vi "System Subpanel.vi"() -> ()   [LabVIEW 2021, in "CIF Manager UI.lvlib"]
uses:
  CIF Manager UI.lvlib
  CIFManagerUI Class/Typedef/New Plugin.ctl
  CIFManagerUI Class/Typedef/Class Data for Manager SubPanel.ctl
  <vilib>/gRPC/LabVIEW gRPC Library/Shared/grpcId.ctl
  <vilib>/CIF Foundation/CIF Core/CIFUI/Typedef/Core UI References.ctl
  <vilib>/CIF Foundation/CIF Core/CIFUI/Typedef/Run Listen Button.ctl
  <vilib>/CIF Foundation/CIF Core/CIFUI/Typedef/SubPanel Events.ctl
  <vilib>/CIF Foundation/CIF Core/CIFUI/Typedef/New Connection Event Data.ctl
  <vilib>/CIF Foundation/CIF Core/CIFUI/Typedef/New Connection Plugin Event Data.ctl
  CIFManagerUI Class/Typedef/Core Manager UI References.ctl
  CIFManagerUI Class/Typedef/Channel Connection.ctl
  CIFManagerUI Class/Typedef/CIF_Manager_UI_Tab.ctl
  CIFManagerUI Class/CIF_Manager_UI.lvclass/CIF_Manager_UI.ctl
  <vilib>/CIF Foundation/CIF Core/CIFUI/CIF_UI.lvclass/CIF_UI.ctl
  <vilib>/CIF Foundation/CIF Core/CIFUI/Utilities/Get Human Readable Error.vi
  <vilib>/CIF Foundation/CIF Utilities/Errors/Append Error Location.vi
  <vilib>/CIF Foundation/CIF Core/CIFUI/Accessors/Read Instrument Studio.vi
  CIFManagerUI Class/CIF_Manager_UI.lvclass
  C:/Program Files/National Instruments/LabVIEW 2021/vi.lib/CIF Foundation/CIF Core/CIFUI/CIF_UI.lvclass
  <vilib>/CIF Foundation/CIF Core/CIFUI/UI Helpers/UI Element Update/Empty Tree by Reference.vi
  CIFManagerUI Class/Manager Functions/SubVIs/Initialize Manager Tab by Reference.vi
  <vilib>/CIF Foundation/CIF Utilities/Errors/Human Readable Error Message.vi
  <vilib>/CIF Foundation/CIF Core/CIFUI/CIF_UI.lvclass
  <vilib>/CIF Foundation/CIF Core/CIFPluginManager/gRPC/CIF_Manager_Client_Wrapper/CIFManagerClientWrapper.lvlib
  <vilib>/gRPC/LabVIEW gRPC Library/grpc-lvsupport-release.lvlib
panel:
  in  "Class Data for Manager SubPanel":T1
  in  "Update Plugin Types":bool
  in  "Load Plugin":bool
  in  "Reset Info":bool
  in  "Get All Info":bool
  in  "Discovered Plugins":string(tree)
  in  "Loaded Plugins":string(tree)
  in  "New Plugin":T6={"Unique Name"="test", "Type"="", "Version (Optional)"="", "Loader (Optional)"=""}
  in  "Abort Plugin":bool
  in  "Plugin to abort":string
  in  "Abort All Plugins":bool
  out "Plugin Metadata":string="\n\n\n\n\n\n\n\n\n\n\n\n\n\n\n\n\n\n\n\n\n\n\n"
  out "Info":string
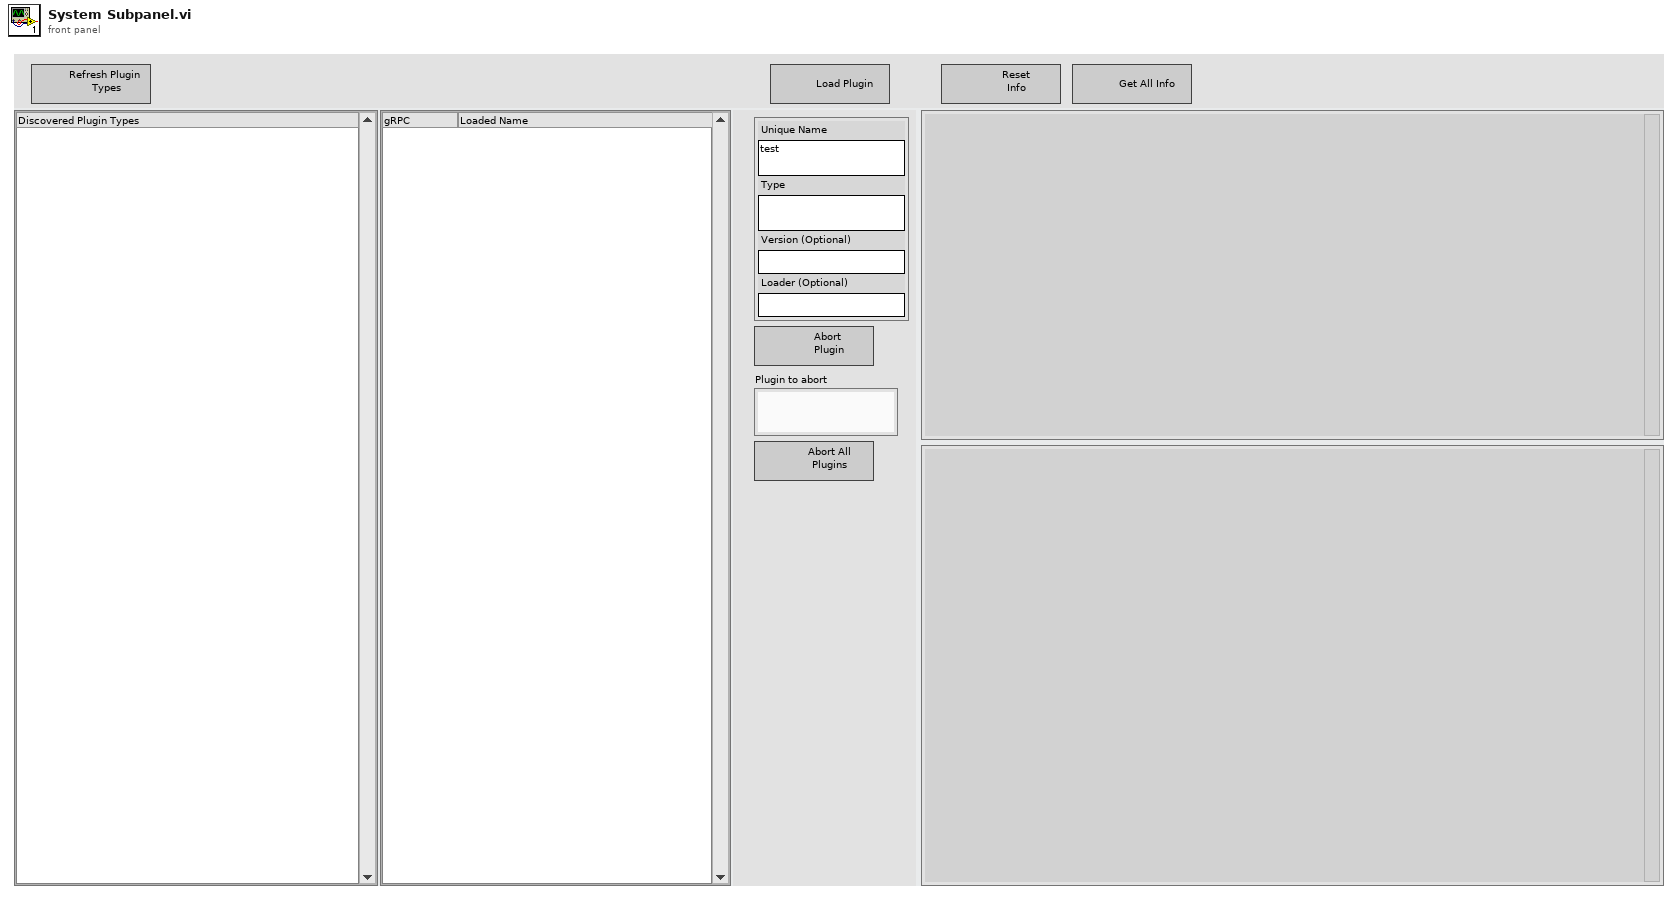
[diagram p1: front panel]
types:
  T1 = typedef "CIF_Manager_UI.lvclass/Class Data for Manager SubPanel.ctl" = cluster{"Class Data for SubPanel":cluster{"IP Address":string, "Manager gRPC ID":T2, "Server Certificate File (.crt)":path, "Connected":bool, "Manager Connection":bool, "Core UI References":T3, "Subpanel Events":T4}, "Manager UI References":T5}
  T2 = typedef "grpc-lvsupport-release.lvlib/grpcId.ctl" = u64
  T3 = typedef "CIF_UI.lvclass/Core UI References.ctl" = cluster{"Plugin Status":refnum<vi>, "Plugin Status Valid":bool, "Connection":refnum<vi>, "Connection Valid":bool, "Exit":refnum<vi>, "Exit Valid":bool, "Run Listen":refnum<vi>, "Run Listen Valid":bool, "Clear Local Error":refnum<vi>, "Clear Local Error Valid":bool, "Local Error":refnum<vi>, "Local Error Valid":bool}
  T4 = typedef "CIF_UI.lvclass/SubPanel Events.ctl" = cluster{"Clear Local Error":refnum<user-event>, "Shutdown":refnum<user-event>, "gRPC Connection":refnum<user-event>, "Plugin Connection":refnum<user-event>}
  T5 = typedef "CIF_Manager_UI.lvclass/Core Manager UI References.ctl" = cluster{"Discovered Plugins":refnum<vi>, "Discovered Plugins Valid":bool, "Loaded Plugins":refnum<vi>, "Loaded Plugins Valid":bool, "Publisher Channels":refnum<vi>, "Publisher Channels Valid":bool, "Subscriber Channels":refnum<vi>, "Subscriber Channels Valid":bool, "Channel Connection":refnum<vi>, "Channel Connection Valid":bool, "New Plugin Load":refnum<vi>, "New Plugin Load Valid":bool, "Errors":refnum<vi>, "Errors Valid":bool, "Plugin to Abort":refnum<vi>, "Plugin to Abort Valid":bool, "CIF Manager Tab":refnum<vi>, "Manger Tab Valid":bool, "System Errors":refnum<vi>, "System Errors Valid":bool, "Plugin Selection":refnum<vi>, "Plugin Selection Valid":bool}
  T6 = typedef "CIF_Manager_UI.lvclass/New Plugin.ctl" = cluster{"Unique Name":string, "Type":string, "Version (Optional)":string, "Loader (Optional)":string}
  T7 = typedef "CIF_Manager_client.lvlib/cif_management_common_PluginMetadata.ctl" = cluster{"description":string, "history":string, "author":string}
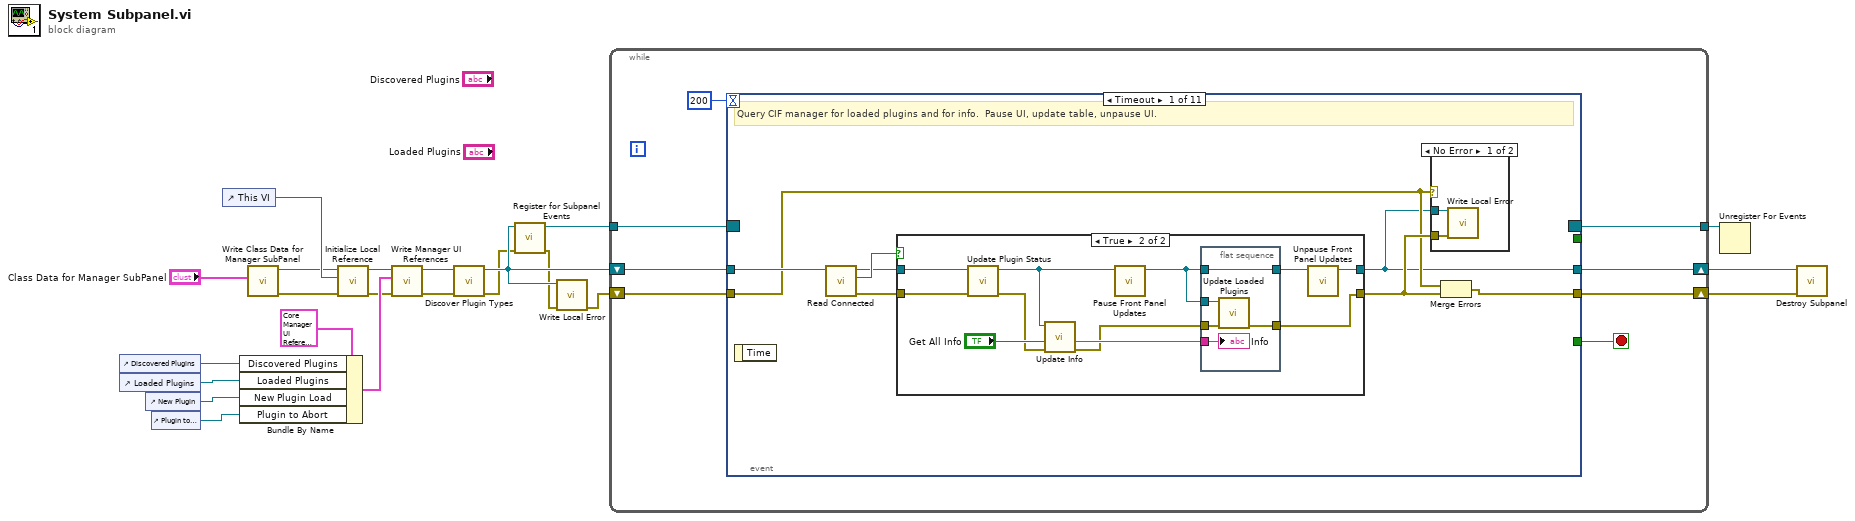
[diagram p0: block diagram]
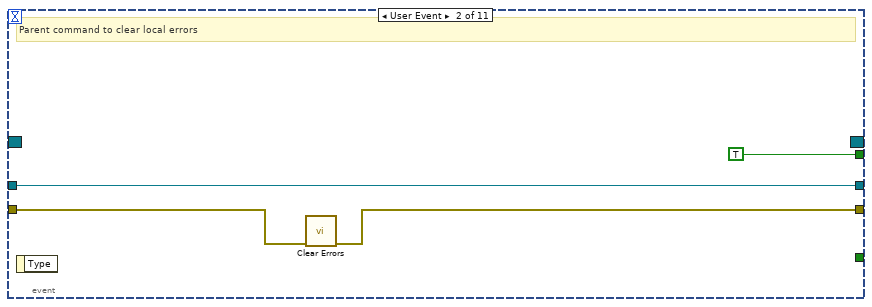
[diagram p4: hidden frame]
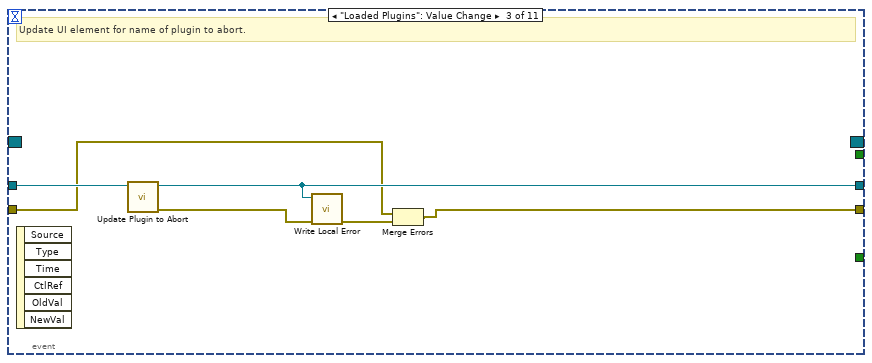
[diagram p5: hidden frame]
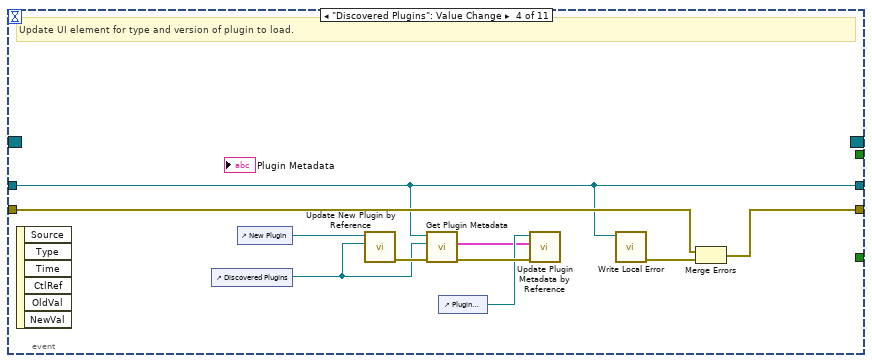
[diagram p6: hidden frame]
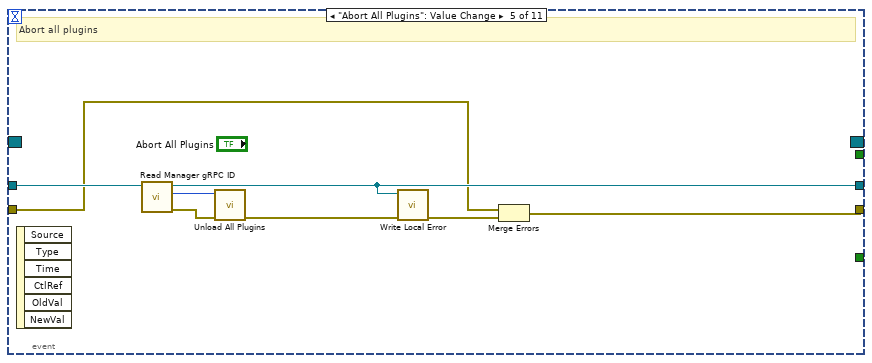
[diagram p7: hidden frame]
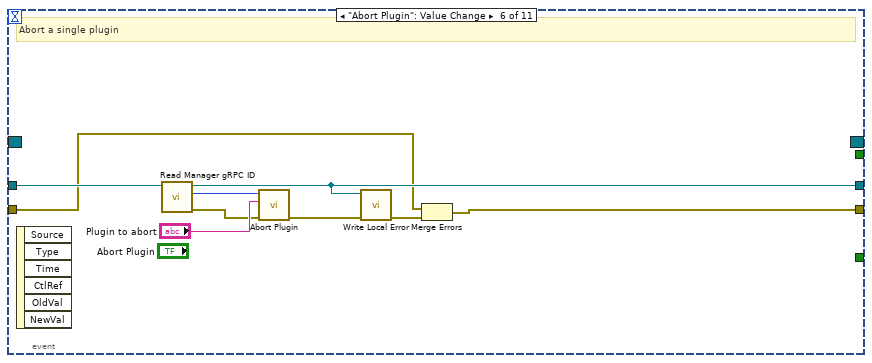
[diagram p8: hidden frame]
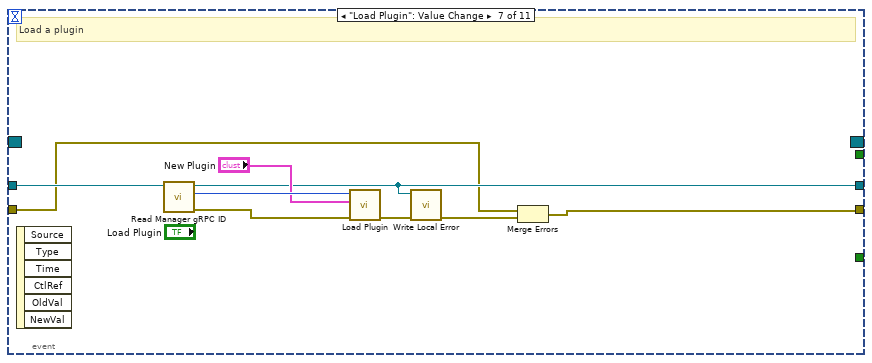
[diagram p9: hidden frame]
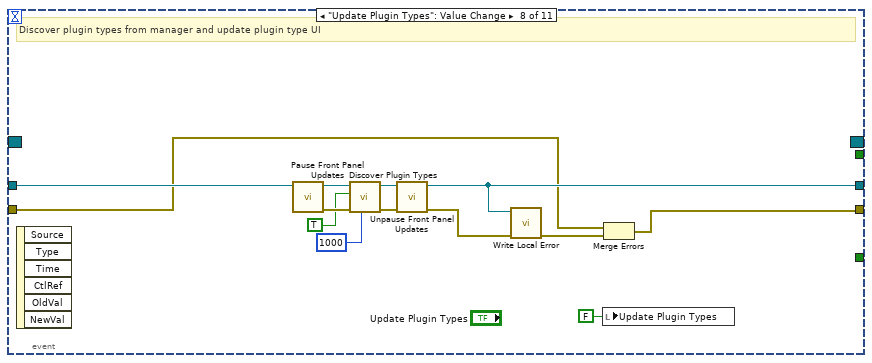
[diagram p10: hidden frame]
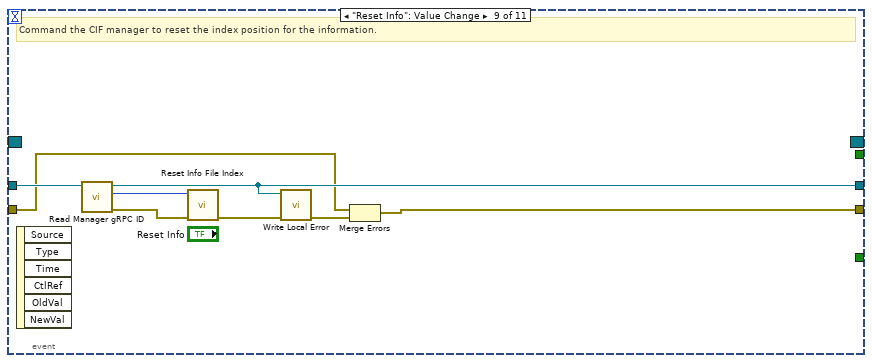
[diagram p11: hidden frame]
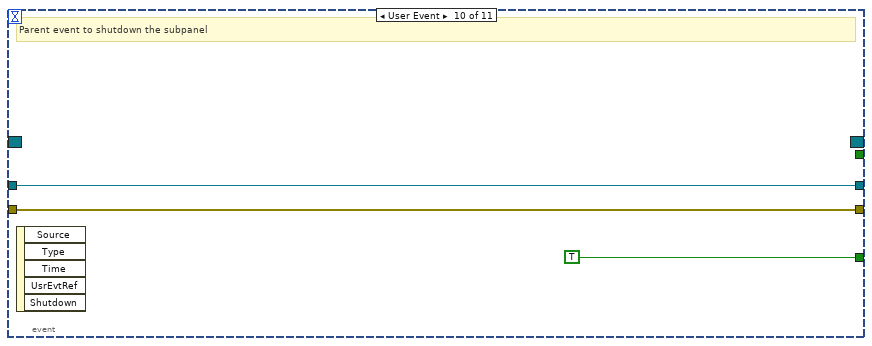
[diagram p12: hidden frame]
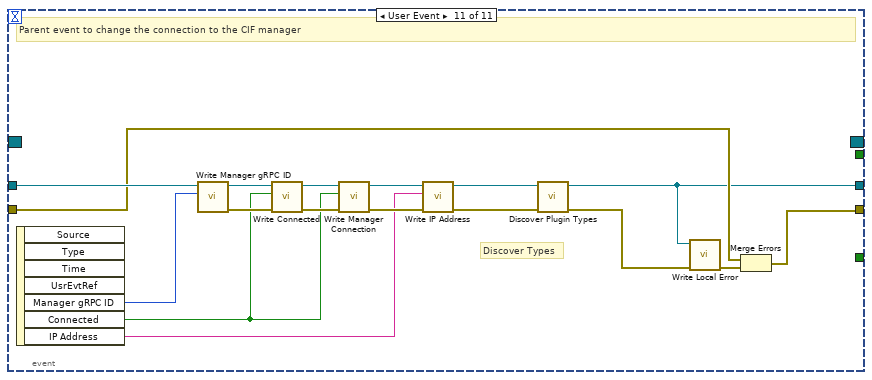
[diagram p13: hidden frame]
diagram:
  n1 = control-ref of="Discovered Plugins"() -> (w22:refnum<vi>)
  n2 = control-ref of="Loaded Plugins"() -> (w21:refnum<vi>)
  n3 = control-ref of="New Plugin"() -> (w20:refnum<vi>)
  n4 = control-ref of="Plugin to abort"() -> (w19:refnum<vi>)
  n5 = control-ref of="This VI"() -> (w17:refnum<vi>)
  n6 = Bundle By Name(cluster=T5 {"Discovered Plugins"=refnum, "Discovered Plugins Valid"=FALSE, "Loaded Plugins"=refnum, "Loaded Plugins Valid"=FALSE, "Publisher Channels"=refnum, "Publisher Channels Valid"=FALSE, "Subscriber Channels"=refnum, "Subscriber Channels Valid"=FALSE, "Channel Connection"=refnum, "Channel Connection Valid"=FALSE, "New Plugin Load"=refnum, "New Plugin Load Valid"=FALSE, "Errors"=refnum, "Errors Valid"=FALSE, "Plugin to Abort"=refnum, "Plugin to Abort Valid"=FALSE, "CIF Manager Tab"=refnum, "Manger Tab Valid"=FALSE, "System Errors"=refnum, "System Errors Valid"=FALSE, "Plugin Selection"=refnum, "Plugin Selection Valid"=FALSE} ("Manager UI References"), "Discovered Plugins"=w22, "Loaded Plugins"=w21, "New Plugin Load"=w20, "Plugin to Abort"=w19) -> (w7:T5)
  n7 = call "Write Class Data for Manager SubPanel.vi"("Class Data for Manager SubPanel"="Class Data for Manager SubPanel") -> ("error out"=w4:errorcluster, "CIF_Manager_UI out"=w3:refnum<class "CIF_Manager_UI.lvclass">)  [unwired: 9 in]
  n8 = call <vilib>:"Initialize Local Reference.vi"("error in (no error)"=w4, "This VI"=w17, "CIF_UI in"=w3) -> ("error out"=w5:errorcluster, "CIF_UI out"=w6:refnum<class "CIF_Manager_UI.lvclass">)  [unwired: 7 in]
  n9 = call "Write Manager UI References.vi"("error in (no error)"=w5, "Manager UI References"=w7, "CIF_UI in"=w6) -> ("error out"=w9:errorcluster, "CIF_UI out"=w8:refnum<class "CIF_Manager_UI.lvclass">)  [unwired: 7 in]
  n10 = call "Discover Plugin Types.vi"("error in (no error)"=w9, "CIF_UI in"=w8) -> ("error out"=w15:errorcluster, "CIF_UI out"=w16:refnum<class "CIF_Manager_UI.lvclass">)  [unwired: 8 in]
  n11 = call <vilib>:"Register for Subpanel Events.vi"("error in (no error)"=w15, "CIF_UI in"=w16) -> ("error out"=w13:errorcluster, "Event Registration Refnum"=w18:refnum<event-registration>)  [unwired: 8 in]
  n12 = call <vilib>:"Write Local Error.vi"("error in (no error)"=w13, "CIF_UI in"=w16) -> ("error out"=w14:errorcluster)  [unwired: 9 in]
  n13 = while {
    shift-right: [w28] -> w12
    shift-left: w16 -> [w27]
    shift-right: [w23] -> w10
    shift-left: w14 -> [w26]
    tunnel: w18 -> [w25]
    tunnel: [w24] -> w11
    stop <- w29 stop-if-true
    n14 = event shown="[0] Timeout" {
      selector: w25 -> [_ _ _ _ _ _ _ _ _ _ _]
      dyn-events: [_ _ _ _ _ _ _ _ _ _ _] -> w24
      timeout: 200 -> [_ _ _ _ _ _ _ _ _ _ _]
      tunnel: [_ _ _ _ _ _ _ _ _ TRUE _] -> w29
      tunnel: w27 -> [w35 w62 w68 w72 w84 w93 w102 w117 w123 w128 w145]
      tunnel: w26 -> [w33 w61 w64 w76 w81 w89 w98 w108 w119 w127 w134]
      tunnel: [w31 w60 w63 w75 w79 w87 w97 w107 w118 w127 w133] -> w23
      tunnel: [w32 w62 w65 w72 w83 w91 w100 w111 w122 w128 w130] -> w28
      tunnel: [_ TRUE _ _ _ _ _ _ _ _ _] -> _
      event Timeout {
        # "Query CIF manager for loaded plugins and for info.  Pause UI, update table, unpause UI."
        n15 = event-data() -> ()  [unwired: 1 in, 1 out]
        n16 = call <vilib>:"Read Connected.vi"("CIF_UI in"=w35) -> ("error out"=w38:errorcluster, "Connected"=w37:bool, "CIF_UI out"=w36:refnum<class "CIF_Manager_UI.lvclass">)  [unwired: 8 in]
        n17 = case shown="True" w37 {
          tunnel: w38 -> [w41 w49]
          tunnel: [w41 w43] -> w34
          tunnel: w36 -> [w42 w50]
          tunnel: [w42 w53] -> w32
          frame False {
          }
          frame True {
            n18 = call <vilib>:"Update Plugin Status.vi"("error in (no error)"=w49, "CIF_UI in"=w50) -> ("error out"=w48:errorcluster, "CIF_UI out"=w47:refnum<class "CIF_Manager_UI.lvclass">)  [unwired: 8 in]
            n19 = call "Update Info.vi"("error in (no error)"=w48, "Get All Info"="Get All Info", "CIF_UI in"=w47) -> ("error out"=w44:errorcluster, "Info"=w51:string)  [unwired: 7 in]
            n20 = call <vilib>:"Pause Front Panel Updates.vi"("CIF_UI in"=w47) -> ("CIF_UI out"=w46:refnum<class "CIF_Manager_UI.lvclass">)  [unwired: 9 in, 1 out]
            n21 = flat-sequence {
              tunnel: w51 -> [w58]
              tunnel: [w57] -> w43
              tunnel: w44 -> [w56]
              tunnel: w46 -> [w55]
              tunnel: w46 -> [w54]
              tunnel: [w54] -> w45
              frame #0 {
                n22 = call "Update Loaded Plugins.vi"("error in (no error)"=w56, "CIF_UI in"=w55) -> ("error out"=w57:errorcluster)  [unwired: 9 in]
                "Info" <- w58
              }
            }
            n23 = call <vilib>:"Unpause Front Panel Updates.vi"("CIF_UI in"=w45) -> ("CIF_UI out"=w53:refnum<class "CIF_Manager_UI.lvclass">)  [unwired: 9 in, 1 out]
          }
        }
        n24 = case shown="No Error" w33 {
          tunnel: w32 -> [w40 _]
          tunnel: w34 -> [w39 _]
          frame No Error {
            n25 = call <vilib>:"Write Local Error.vi"("error in (no error)"=w39, "CIF_UI in"=w40) -> ()  [unwired: 9 in, 1 out]
          }
          frame Error {
          }
        }
        n26 = Merge Errors(w33, w34) -> (w31:errorcluster)
      }
      event User Event {
        # "Parent command to clear local errors"
        n27 = event-data() -> ()  [unwired: 1 in, 1 out]
        n28 = call <vilib>:"Clear Errors.vi"("error in (no error)"=w61) -> ("error out"=w60:errorcluster)  [unwired: 5 in, 1 out]
      }
      event "Loaded Plugins": Value Change {
        # "Update UI element for name of plugin to abort."
        n29 = event-data() -> ()  [unwired: 1 in, 6 out]
        n30 = call "Update Plugin to Abort.vi"("CIF_UI in"=w68) -> ("error out"=w67:errorcluster, "CIF_UI out"=w65:refnum<class "CIF_Manager_UI.lvclass">)  [unwired: 9 in]
        n31 = call <vilib>:"Write Local Error.vi"("error in (no error)"=w67, "CIF_UI in"=w65) -> ("error out"=w66:errorcluster)  [unwired: 9 in]
        n32 = Merge Errors(w64, w66) -> (w63:errorcluster)
      }
      event "Discovered Plugins": Value Change {
        # "Update UI element for type and version of plugin to load."
        n33 = event-data() -> ()  [unwired: 1 in, 6 out]
        n34 = control-ref of="Discovered Plugins"() -> (w73:refnum<vi>)
        n35 = control-ref of="New Plugin"() -> (w78:refnum<vi>)
        n36 = call "Update New Plugin by Reference.vi"("Plugin Types Tree"=w73, "New Plugin Control"=w78) -> ("error out"=w74:errorcluster)  [unwired: 9 in]
        n37 = call "Get Plugin Metadata.vi"("error in (no error)"=w74, "Plugin Types Tree"=w73, "CIF_UI in"=w72) -> ("error out"=w71:errorcluster, "plugin_metadata"=w69:T7)  [unwired: 7 in]
        n38 = control-ref of="Plugin Metadata"() -> (w70:refnum<vi>)
        n39 = call "Update Plugin Metadata by Reference.vi"("error in (no error)"=w71, "plugin_metadata"=w69, "Metadata"=w70) -> ()  [unwired: 8 in, 1 out]
        n40 = call <vilib>:"Write Local Error.vi"("CIF_UI in"=w72) -> ("error out"=w77:errorcluster)  [unwired: 10 in]
        n41 = Merge Errors(w76, w77) -> (w75:errorcluster)
      }
      event "Abort All Plugins": Value Change {
        # "Abort all plugins"
        n42 = event-data() -> ()  [unwired: 1 in, 6 out]
        n43 = call <vilib>:"Read Manager gRPC ID.vi"("CIF_UI in"=w84) -> ("error out"=w85:errorcluster, "Manager gRPCid"=w86:T2, "CIF_UI out"=w83:refnum<class "CIF_Manager_UI.lvclass">)  [unwired: 8 in]
        n44 = call <vilib>:"Unload All Plugins.vi"("error in"=w85, "gRPC ID in"=w86) -> ("error out"=w80:errorcluster)  [unwired: 8 in, 1 out]
        n45 = call <vilib>:"Write Local Error.vi"("error in (no error)"=w80, "CIF_UI in"=w83) -> ("error out"=w82:errorcluster)  [unwired: 9 in]
        n46 = Merge Errors(w81, w82) -> (w79:errorcluster)
      }
      event "Abort Plugin": Value Change {
        # "Abort a single plugin"
        n47 = event-data() -> ()  [unwired: 1 in, 6 out]
        n48 = call <vilib>:"Read Manager gRPC ID.vi"("CIF_UI in"=w93) -> ("error out"=w92:errorcluster, "Manager gRPCid"=w95:T2, "CIF_UI out"=w91:refnum<class "CIF_Manager_UI.lvclass">)  [unwired: 8 in]
        n49 = call <vilib>:"Abort Plugin.vi"("error in"=w92, "plugin_name"="Plugin to abort", "gRPC ID in"=w95) -> ("error out"=w88:errorcluster)  [unwired: 7 in, 1 out]
        n50 = call <vilib>:"Write Local Error.vi"("error in (no error)"=w88, "CIF_UI in"=w91) -> ("error out"=w90:errorcluster)  [unwired: 9 in]
        n51 = Merge Errors(w89, w90) -> (w87:errorcluster)
      }
      event "Load Plugin": Value Change {
        # "Load a plugin"
        n52 = event-data() -> ()  [unwired: 1 in, 6 out]
        n53 = call <vilib>:"Read Manager gRPC ID.vi"("CIF_UI in"=w102) -> ("error out"=w103:errorcluster, "Manager gRPCid"=w104:T2, "CIF_UI out"=w100:refnum<class "CIF_Manager_UI.lvclass">)  [unwired: 8 in]
        n54 = call <vilib>:"Load Plugin.vi"("error in"=w103, "New Plugin"="New Plugin", "gRPC ID in"=w104) -> ("error out"=w96:errorcluster)  [unwired: 7 in, 1 out]
        n55 = call <vilib>:"Write Local Error.vi"("error in (no error)"=w96, "CIF_UI in"=w100) -> ("error out"=w99:errorcluster)  [unwired: 9 in]
        n56 = Merge Errors(w98, w99) -> (w97:errorcluster)
      }
      event "Update Plugin Types": Value Change {
        # "Discover plugin types from manager and update plugin type UI"
        n57 = event-data() -> ()  [unwired: 1 in, 6 out]
        n58 = call <vilib>:"Pause Front Panel Updates.vi"("CIF_UI in"=w117) -> ("error out"=w116:errorcluster, "CIF_UI out"=w115:refnum<class "CIF_Manager_UI.lvclass">)  [unwired: 9 in]
        n59 = call "Discover Plugin Types.vi"("timeout (ms)"=1000, "error in (no error)"=w116, "reload"=TRUE, "CIF_UI in"=w115) -> ("error out"=w113:errorcluster, "CIF_UI out"=w114:refnum<class "CIF_Manager_UI.lvclass">)  [unwired: 6 in]
        n60 = call <vilib>:"Unpause Front Panel Updates.vi"("error in (no error)"=w113, "CIF_UI in"=w114) -> ("error out"=w110:errorcluster, "CIF_UI out"=w111:refnum<class "CIF_Manager_UI.lvclass">)  [unwired: 8 in]
        n61 = call <vilib>:"Write Local Error.vi"("error in (no error)"=w110, "CIF_UI in"=w111) -> ("error out"=w109:errorcluster)  [unwired: 9 in]
        n62 = local write "Update Plugin Types"(FALSE ("Update Plugin Types")) -> ()
        n63 = Merge Errors(w108, w109) -> (w107:errorcluster)
      }
      event "Reset Info": Value Change {
        # "Command the CIF manager to reset the index position for the information."
        n64 = event-data() -> ()  [unwired: 1 in, 6 out]
        n65 = call <vilib>:"Read Manager gRPC ID.vi"("CIF_UI in"=w123) -> ("error out"=w124:errorcluster, "Manager gRPCid"=w125:T2, "CIF_UI out"=w122:refnum<class "CIF_Manager_UI.lvclass">)  [unwired: 8 in]
        n66 = call <vilib>:"Reset Info File Index.vi"("error in"=w124, "gRPC ID in"=w125) -> ("error out"=w121:errorcluster)  [unwired: 8 in, 1 out]
        n67 = call <vilib>:"Write Local Error.vi"("error in (no error)"=w121, "CIF_UI in"=w122) -> ("error out"=w120:errorcluster)  [unwired: 9 in]
        n68 = Merge Errors(w119, w120) -> (w118:errorcluster)
      }
      event User Event {
        # "Parent event to shutdown the subpanel"
        n69 = event-data() -> ()  [unwired: 1 in, 5 out]
      }
      event User Event {
        # "Discover Types"
        # "Parent event to change the connection to the CIF manager"
        n70 = event-data() -> ("Manager gRPC ID"=w138:T2, "Connected"=w137:bool, "IP Address"=w136:string)  [unwired: 1 in, 4 out]
        n71 = call <vilib>:"Write Manager gRPC ID.vi"("gRPCid"=w138, "CIF_UI in"=w145) -> ("error out"=w143:errorcluster, "CIF_UI out"=w144:refnum<class "CIF_Manager_UI.lvclass">)  [unwired: 8 in]
        n72 = call <vilib>:"Write Connected.vi"("error in (no error)"=w143, "Connected"=w137, "CIF_UI in"=w144) -> ("error out"=w141:errorcluster, "CIF_UI out"=w142:refnum<class "CIF_Manager_UI.lvclass">)  [unwired: 7 in]
        n73 = call <vilib>:"Write Manager Connection.vi"("error in (no error)"=w141, "Manager Connection"=w137, "CIF_UI in"=w142) -> ("error out"=w139:errorcluster, "CIF_UI out"=w140:refnum<class "CIF_Manager_UI.lvclass">)  [unwired: 7 in]
        n74 = call <vilib>:"Write IP Address.vi"("error in (no error)"=w139, "IP Address"=w136, "CIF_UI in"=w140) -> ("error out"=w131:errorcluster, "CIF_UI out"=w132:refnum<class "CIF_Manager_UI.lvclass">)  [unwired: 7 in]
        n75 = call "Discover Plugin Types.vi"("error in (no error)"=w131, "CIF_UI in"=w132) -> ("error out"=w129:errorcluster, "CIF_UI out"=w130:refnum<class "CIF_Manager_UI.lvclass">)  [unwired: 8 in]
        n76 = call <vilib>:"Write Local Error.vi"("error in (no error)"=w129, "CIF_UI in"=w130) -> ("error out"=w135:errorcluster)  [unwired: 9 in]
        n77 = Merge Errors(w134, w135) -> (w133:errorcluster)
      }
    }
  }
  n78 = Unregister For Events(event registration refnum=w11) -> ()  [unwired: 1 in, 1 out]
  n79 = call <vilib>:"Destroy Subpanel.vi"("error in (no error)"=w10, "CIF_UI in"=w12) -> ()  [unwired: 8 in, 2 out]
